vi "Connect.vi"(8 "error in (no error)":errorcluster, 11 "2230G in":refnum<class "2230G.lvclass">) -> (0 "error out":errorcluster, 3 "2230G out":refnum<class "2230G.lvclass">)   [LabVIEW 2018, in "2230G.lvlib" / "2230G.lvclass"]
uses:
  2230G.lvclass
  PPLs/Power Supply/Parent/Power_Supply.lvlibp/Power Supply.lvclass
  <instrlib>/Keithley KE22xx Series/Keithley KE22xx Series.lvlib
  C:/Projects/LabVIEW/PPLs/Power Supply/Parent/Power_Supply.lvlibp/Power Supply.lvclass
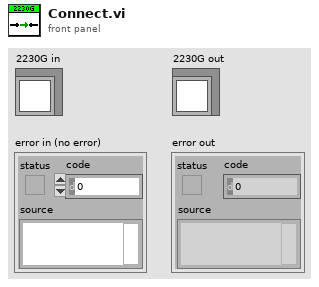
[diagram p1: front panel]
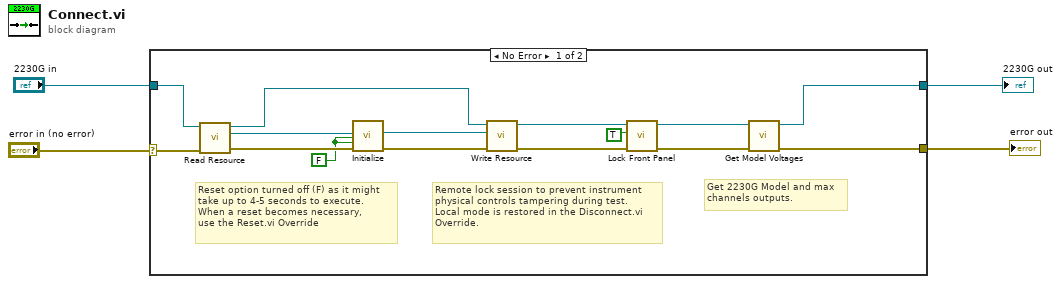
[diagram p0: block diagram]
diagram:
  n1 = case shown="No Error" "error in (no error)" {
    selector: "error in (no error)" -> [w19 w20]
    tunnel: "2230G in" -> [w18 w21]
    tunnel: [w8 w21] -> w2
    tunnel: [w6 w20] -> w1
    frame No Error {
      w5 = FALSE ("Reset (True)")
      # "Get 2230G Model and max\nchannels outputs."
      # "Remote lock session to prevent instrument\nphysical controls tampering during test.\nLocal mode is restored in the Disconnect.vi\nOverride."
      # "Reset option turned off (F) as it might\ntake up to 4-5 seconds to execute. \nWhen a reset becomes necessary, \nuse the Reset.vi Override"
      n2 = call "Read Resource.vi"("error in"=w19, "Power Supply in"=w18) -> ("error out"=w16:errorcluster, "Resource"=w17:refnum<visa-resource-name>, "Power Supply out"=w15:refnum<class "2230G.lvclass">)  [unwired: 7 in]
      n3 = call <instrlib>:"Initialize.vi"("error in (no error)"=w16, "Reset (True)"=w5, "ID Query (True)"=w5, "VISA resource name"=w17) -> ("error out"=w13:errorcluster, "VISA resource name out"=w14:refnum<visa-resource-name>)  [unwired: 6 in]
      n4 = call "Write Resource.vi"("error in"=w13, "Resource"=w14, "Power Supply in"=w15) -> ("error out"=w12:errorcluster, "Power Supply out"=w11:refnum<class "2230G.lvclass">)  [unwired: 7 in]
      n5 = call-dynamic "Lock Front Panel.vi"("error in (no error)"=w12, "Lock?"=TRUE, "2230G in"=w11) -> ("error out"=w7:errorcluster, "2230G out"=w9:refnum<class "2230G.lvclass">)  [unwired: 7 in]
      n6 = call "Get Model Voltages.vi"("error in (no error)"=w7, "2230G in"=w9) -> ("error out"=w6:errorcluster, "2230G out"=w8:refnum<class "2230G.lvclass">)  [unwired: 8 in]
    }
    frame Error {
    }
  }
  "error out" <- w1
  "2230G out" <- w2
